vi "EMV No Flow Slope Check.vi"(8 "error in (no error)":errorcluster, 10 "Detection Slope":dbl=0.2 format="%#_13g", 11 "T7 History Output":dbl[](array[numeric])) -> (0 "error out":errorcluster, 2 "Detection?":bool, 3 "Slope History":dbl[](array[numeric]))   [LabVIEW 2016]
uses:
  <vilib>/Analysis/baseanly.llb/Mean (DBL).vi
  <vilib>/Analysis/NI_AALBase.lvlib
panel:
  out "T7 Rise Acceleration Chart":dbl(graph)
  out "T7 Rise Acceleration":dbl[](array[numeric])
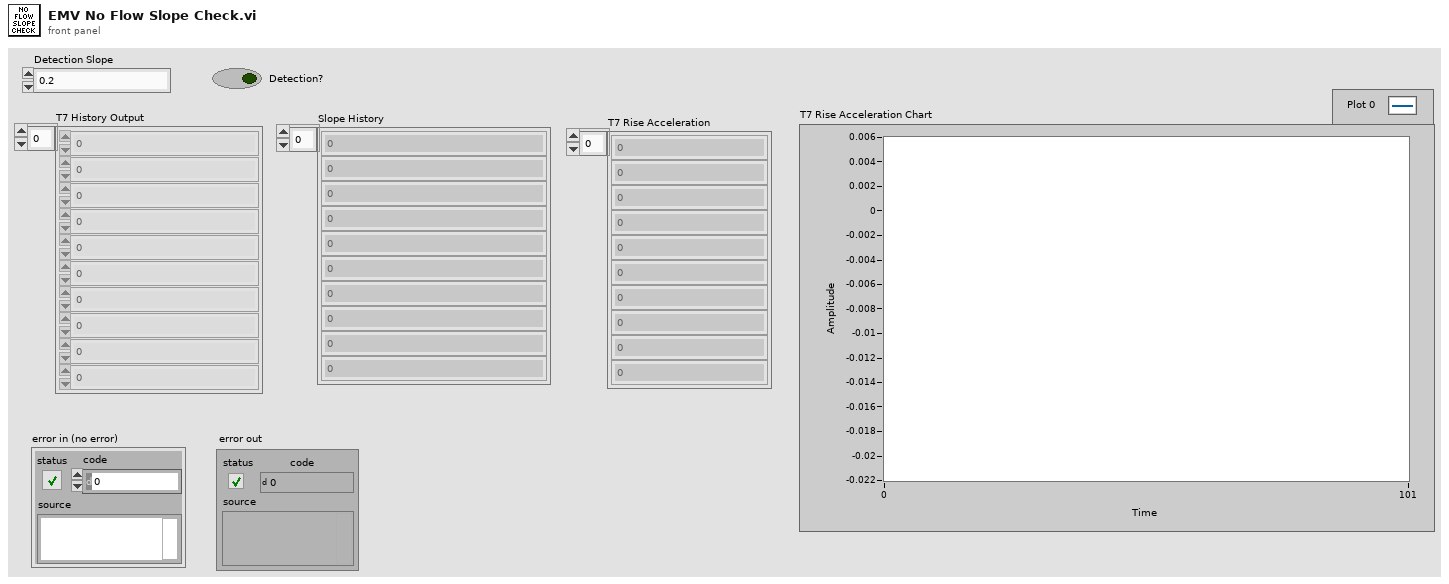
[diagram p1: front panel]
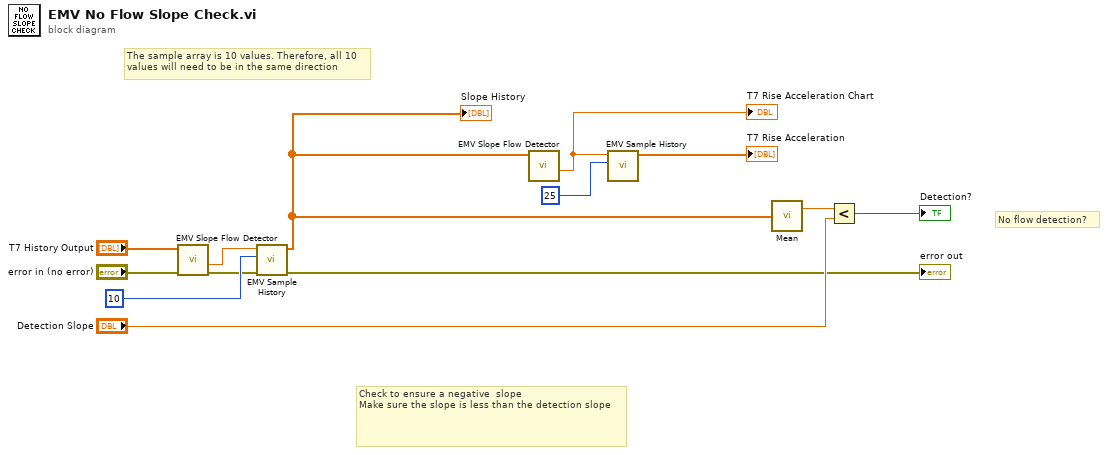
[diagram p0: block diagram]
diagram:
  # "No flow detection?"
  # "Check to ensure a negative  slope \nMake sure the slope is less than the detection slope"
  # "The sample array is 10 values. Therefore, all 10\nvalues will need to be in the same direction"
  n1 = call "EMV Slope Flow Detector.vi"("error in (no error)"="error in (no error)", "Current T6 Temperatures in"="T7 History Output") -> ("error out"=w5:errorcluster, "slope"=w6:dbl)  [unwired: 5 in, 3 out]
  n2 = call "EMV Sample History.vi"("error in (no error)"=w5, "length"=10, "T6 Temp"=w6) -> ("error out"=→"error out":errorcluster, "T6 History"=w4:dbl[])  [unwired: 7 in]
  "Slope History" <- w4
  n3 = call "EMV Slope Flow Detector.vi"("Current T6 Temperatures in"=w4) -> ("slope"=w1:dbl)  [unwired: 6 in, 4 out]
  "T7 Rise Acceleration Chart" <- w1
  n4 = call "EMV Sample History.vi"("length"=25, "T6 Temp"=w1) -> ("T6 History"=→"T7 Rise Acceleration":dbl[])  [unwired: 8 in, 1 out]
  n5 = call-poly <vilib>:"Mean.vi"("X"=w4) -> ("mean"=w8:dbl)  [unwired: 1 out]
  n6 = Less?(x=w8, y="Detection Slope") -> (x < y?=→"Detection?":bool)
